vi "CAN Jaguar Set Output.vi"(8 "error in (no error)":errorcluster, 9 "Sync group bit mask":u8, 10 "Output Set Point":dbl, 11 "CAN Jaguar Ref":T1={"Device Number"=0, "Control Mode"=enum."Percent VBus", "Inverted"=FALSE, "Semaphore"=refnum, "Max Vout"=12.0, "DevStatus"={"status"=FALSE, "code"=0, "source"=""}}) -> (0 "error out":errorcluster, 3 "CAN Jaguar Ref Out":T1={"Device Number"=0, "Control Mode"=enum."Percent VBus", "Inverted"=FALSE, "Semaphore"=refnum, "Max Vout"=12.0, "DevStatus"={"status"=FALSE, "code"=0, "source"=""}})   [LabVIEW 2009, in "CAN.lvlib"]
uses:
  CAN.lvlib
  SubVIs/CAN Jaguar Ref.ctl
  SubVIs/CAN Jaguar Control Mode.ctl
  SubVIs/CAN Token Message IDs.ctl
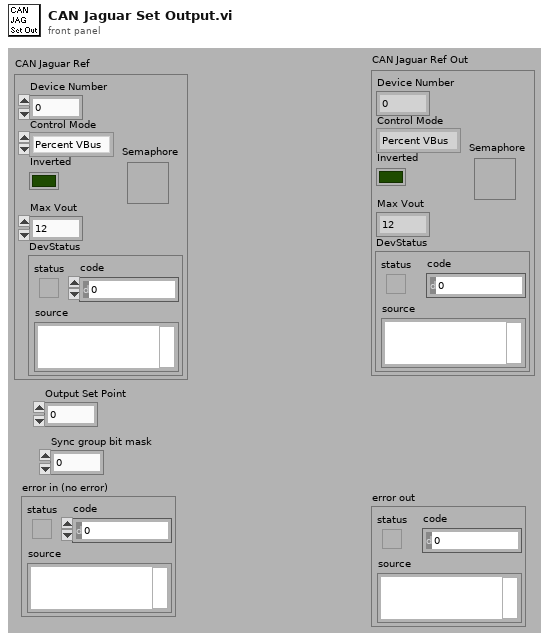
[diagram p1: front panel]
types:
  T1 = typedef "CAN.lvlib/CAN Jaguar Ref.ctl" = cluster{"Device Number":u8, "Control Mode":T2, "Inverted":bool, "Semaphore":T3, "Max Vout":dbl, "DevStatus":errorcluster}
  T2 = typedef "CAN.lvlib/CAN Jaguar Control Mode.ctl" = enum16{"Percent VBus", "Speed", "Position", "Current"}
  T3 = typedef "Semaphore RefNum" = refnum<k1>
  T4 = enum16{"big-endian, network order", "native, host order", "little-endian"}
  T5 = typedef "CAN.lvlib/CAN Token Message IDs.ctl" = u32
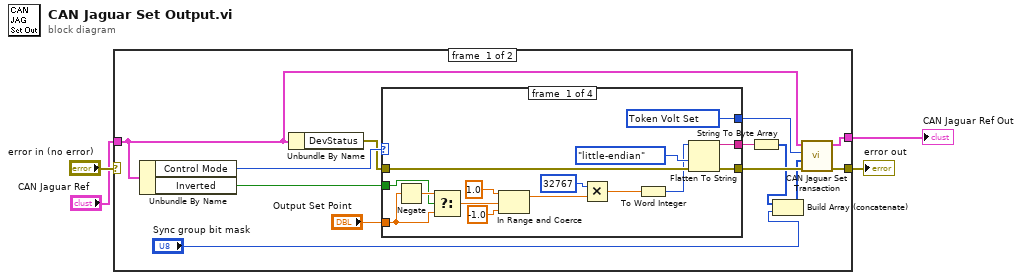
[diagram p0: block diagram]
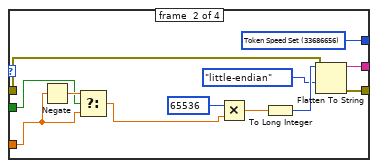
[diagram p2: hidden frame]
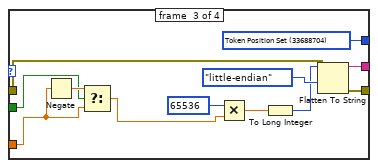
[diagram p3: hidden frame]
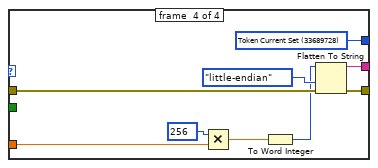
[diagram p4: hidden frame]
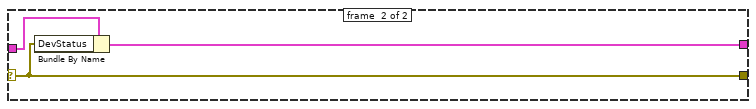
[diagram p5: hidden frame]
diagram:
  n1 = case shown="No Error" "error in (no error)" {
    selector: "error in (no error)" -> [_ w66]
    tunnel: [w10 w66] -> w4
    tunnel: [w11 w67] -> w2
    tunnel: "CAN Jaguar Ref" -> [w8 w68]
    frame #0 {
      n2 = Unbundle By Name(w8) -> ("Control Mode"=w17:T2, "Inverted"=w14:bool)
      n3 = Unbundle By Name(w8) -> ("DevStatus"=w9:errorcluster)
      n4 = case shown="\"Position\"" w17 {
        tunnel: [w32 w44 w49 w65] -> w12
        tunnel: "Output Set Point" -> [w20 w34 w46 w59]
        tunnel: w9 -> [w28 w41 w53 w63]
        tunnel: [w27 w40 w52 w62] -> w13
        tunnel: [w22 w39 w54 w61] -> w15
        tunnel: w14 -> [w19 w33 w45 _]
        frame #0 {
          w32 = T5 33685632 items=["Token Volt Enable"=33685504, "Token Volt Set"=33685632, "Token Speed Enable"=33686528, "Token Speed Set"=33686656, "Token Position Enable"=33688576, "Token Position Set"=33688704, "Token Current Enable"=33689600, "Token Current Set"=33689728] ("CAN Token Message IDs")
          n5 = Negate(x=w20) -> (-x=w21:dbl)
          n6 = Select(t=w21, s=w19, f=w20) -> (s? t:f=w18:dbl)
          n7 = In Range and Coerce(upper limit=1.0, x=w18, lower limit=-1.0) -> (coerced(x)=w26:dbl)  [unwired: 1 out]
          n8 = Multiply(x=i16 32767, y=w26) -> (x*y=w24:dbl)
          n9 = To Word Integer(number=w24) -> (16bit integer=w23:i16)
          n10 = Flatten To String(anything=w23, byte order (0:big-endian, network order)=T4."little-endian", error in (no error)=w28) -> (data string=w22:string, error out=w27:errorcluster)  [unwired: 2 out]
        }
        frame #1 {
          w44 = T5 33686656 items=["Token Volt Enable"=33685504, "Token Volt Set"=33685632, "Token Speed Enable"=33686528, "Token Speed Set"=33686656, "Token Position Enable"=33688576, "Token Position Set"=33688704, "Token Current Enable"=33689600, "Token Current Set"=33689728] ("CAN Token Message IDs")
          n11 = Negate(x=w34) -> (-x=w36:dbl)
          n12 = Select(t=w36, s=w33, f=w34) -> (s? t:f=w35:dbl)
          n13 = Multiply(x=u32 65536, y=w35) -> (x*y=w37:dbl)
          n14 = To Long Integer(number=w37) -> (32bit integer=w43:i32)
          n15 = Flatten To String(anything=w43, byte order (0:big-endian, network order)=T4."little-endian", error in (no error)=w41) -> (data string=w39:string, error out=w40:errorcluster)  [unwired: 2 out]
        }
        frame #2 {
          w49 = T5 33688704 items=["Token Volt Enable"=33685504, "Token Volt Set"=33685632, "Token Speed Enable"=33686528, "Token Speed Set"=33686656, "Token Position Enable"=33688576, "Token Position Set"=33688704, "Token Current Enable"=33689600, "Token Current Set"=33689728] ("CAN Token Message IDs")
          n16 = Negate(x=w46) -> (-x=w48:dbl)
          n17 = Select(t=w48, s=w45, f=w46) -> (s? t:f=w47:dbl)
          n18 = Multiply(x=u32 65536, y=w47) -> (x*y=w50:dbl)
          n19 = To Long Integer(number=w50) -> (32bit integer=w55:i32)
          n20 = Flatten To String(anything=w55, byte order (0:big-endian, network order)=T4."little-endian", error in (no error)=w53) -> (data string=w54:string, error out=w52:errorcluster)  [unwired: 2 out]
        }
        frame #3 {
          w65 = T5 33689728 items=["Token Volt Enable"=33685504, "Token Volt Set"=33685632, "Token Speed Enable"=33686528, "Token Speed Set"=33686656, "Token Position Enable"=33688576, "Token Position Set"=33688704, "Token Current Enable"=33689600, "Token Current Set"=33689728] ("CAN Token Message IDs")
          n21 = Multiply(x=u32 256, y=w59) -> (x*y=w58:dbl)
          n22 = To Word Integer(number=w58) -> (16bit integer=w60:i16)
          n23 = Flatten To String(anything=w60, byte order (0:big-endian, network order)=T4."little-endian", error in (no error)=w63) -> (data string=w61:string, error out=w62:errorcluster)  [unwired: 2 out]
        }
      }
      n24 = String To Byte Array(string=w15) -> (unsigned byte array=w6:u8[])
      n25 = Build Array (concatenate)(w6, "Sync group bit mask") -> (w5:u8[])
      n26 = call "CAN Jaguar Set Transaction.vi"("error in"=w13, "Data"=w5, "Message ID"=w12, "CAN Jaguar Ref"=w8) -> ("error out"=w10:errorcluster, "CAN Jaguar Ref Out"=w11:T1)  [unwired: 6 out]
    }
    frame #1 {
      n27 = Bundle By Name(cluster=w68, "DevStatus"=w66) -> (w67:T1)
    }
  }
  "CAN Jaguar Ref Out" <- w2
  "error out" <- w4
